vi "Test Sync.vi"() -> ()   [LabVIEW 2014, in "SyncPlugins.lvlib" / "NiPxi6682.lvclass"]
uses:
  NiPxi6682.lvclass
  NiPxi6682.lvclass/NiPxi6682.ctl
  SyncPluginBase/SyncPluginBase.lvclass/SyncPluginBase.ctl
  SyncPluginBase/Accessors/Read Locked.vi
  SyncPluginBase/Accessors/Read LostLock.vi
  Accessors/Write 1PPS.vi
  Accessors/Write PgmPPS.vi
  Accessors/Write PgmPPSFreq.vi
  Accessors/Write DdsFreq.vi
panel:
  out "Status":string
  in  "stop":bool
  out "Time Ref Offset (ns)":dbl format="%#_12f"
  out "LostLock":bool
  out "Locked":bool
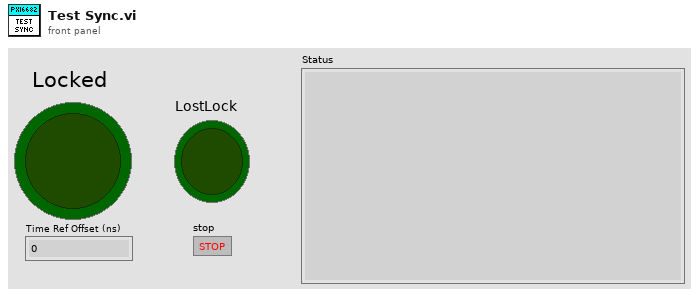
[diagram p1: front panel]
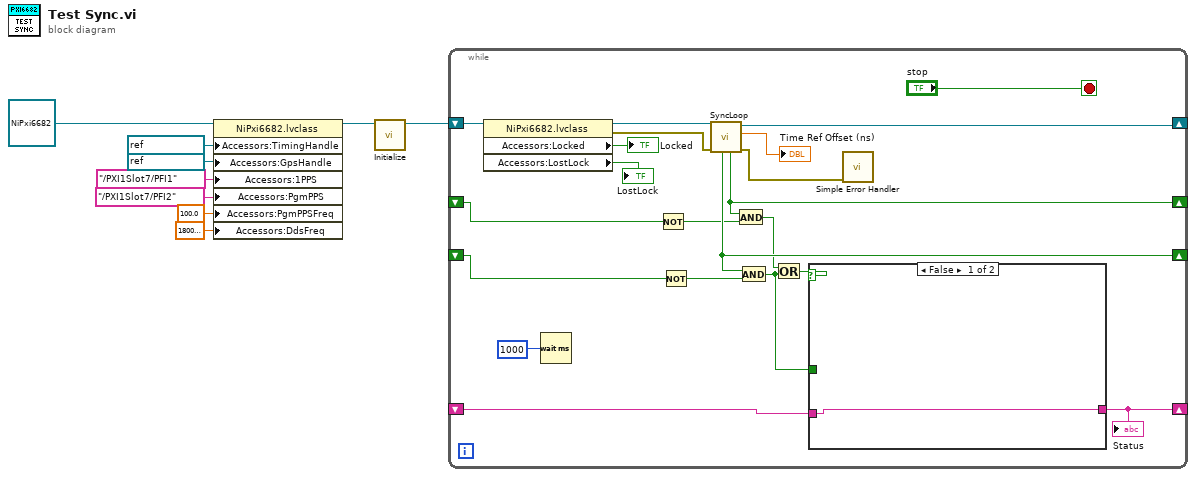
[diagram p0: block diagram]
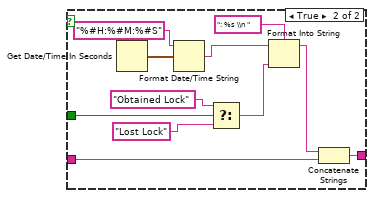
[diagram p2: hidden frame]
diagram:
  n1 = property class="NiPxi6682.lvclass"(reference=refnum<class "NiPxi6682.lvclass"> refnum ("SyncPlugins.lvlib:NiPxi6682.lvclass"), "Accessors:TimingHandle"=refnum<k15> "PXI1Slot4" ("TimingHandle"), "Accessors:GpsHandle"=refnum<k15> "PXI1Slot7" ("GpsHandle"), "Accessors:1PPS"=tag "/PXI1Slot7/PFI1" ("1PPS"), "Accessors:PgmPPS"=tag "/PXI1Slot7/PFI2" ("PgmPPS"), "Accessors:PgmPPSFreq"=100.0 ("PgmPPSFreq"), "Accessors:DdsFreq"=18000000.0 ("DdsFreq")) -> (reference out=w2:refnum<class "NiPxi6682.lvclass">)  [unwired: 1 in, 1 out]
  n2 = call-dynamic "Initialize.vi"("NiPxi6682 in"=w2) -> ("NiPxi6682 out"=w1:refnum<class "NiPxi6682.lvclass">)  [unwired: 9 in, 1 out]
  n3 = while {
    shift-right: [w23] -> _
    shift-left: w1 -> [w30]
    shift-right: [w18] -> _
    shift-left: _ -> [w17]
    shift-right: [w20] -> _
    shift-left: _ -> [w19]
    shift-right: [w11] -> _
    shift-left: _ -> [w10]
    stop <- "stop" stop-if-true
    n4 = property class="NiPxi6682.lvclass"(reference=w30) -> (reference out=w29:refnum<class "NiPxi6682.lvclass">, error out=w25:errorcluster, "Accessors:Locked"=→"Locked":bool, "Accessors:LostLock"=→"LostLock":bool)  [unwired: 1 in]
    n5 = Wait (ms)(milliseconds to wait=u32 1000) -> ()  [unwired: 1 out]
    n6 = Not(x=w19) -> (.not. x?=w13:bool)
    n7 = Not(x=w17) -> (.not. x?=w14:bool)
    n8 = call-dynamic "SyncLoop.vi"("error in (no error)"=w25, "NiPxi6682 in"=w29) -> ("error out"=w24:errorcluster, "Time Ref Offset (ns)"=→"Time Ref Offset (ns)":dbl, "NiPxi6682 out"=w23:refnum<class "NiPxi6682.lvclass">, "Lost Lock"=w20:bool, "ObtainLock"=w18:bool)  [unwired: 5 in]
    n9 = And(x=w20, y=w13) -> (x .and. y?=w16:bool)
    n10 = And(x=w18, y=w14) -> (x .and. y?=w12:bool)
    n11 = Or(x=w16, y=w12) -> (x .or. y?=w15:bool)
    n12 = case shown="False" w15 {
      tunnel: w12 -> [_ w40]
      tunnel: [w31 w33] -> w11
      tunnel: w10 -> [w31 w32]
      frame False {
      }
      frame True {
        n13 = Get Date/Time In Seconds() -> (seconds since 1Jan1904=w39:timestamp)
        n14 = Format Date/Time String(time format string (%c)="%#H:%#M:%#S", seconds (now)=w39) -> (date/time string=w36:string)  [unwired: 1 in]
        n15 = Select(t="Obtained Lock", s=w40, f="Lost Lock") -> (s? t:f=w35:string)
        n16 = Format Into String(format string=": %s \\n ", initial string=w36, w35) -> (resulting string=w34:string)  [unwired: 1 in, 1 out]
        n17 = Concatenate Strings(w34, w32) -> (w33:string)
      }
    }
    "Status" <- w11
    n18 = call <vilib>:"Simple Error Handler.vi"("error in (no error)"=w24) -> ()  [unwired: 4 in, 5 out]
  }
